vi "Example.vi"() -> ()   [LabVIEW 2020, in "lvpptx.lvlib"]
uses:
  lvpptx.lvlib
  Font.ctl
  Textframe Resize Policy.ctl
  Slide Type.ctl
  Position.ctl
  Size.ctl
panel:
  in  "Text":string
  in  "Text formatting":T1={"Font"="Arial", "Size"=18.0, "Italic"=FALSE, "Bold"=FALSE, "Underline"=FALSE, "Color"=0}
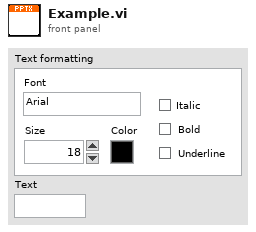
[diagram p1: front panel]
types:
  T1 = typedef "lvpptx.lvlib/Font.ctl" = cluster{"Font":string, "Size":dbl, "Italic":bool, "Bold":bool, "Underline":bool, "Color":u32}
  T2 = typedef "lvpptx.lvlib/Size.ctl" = cluster{"W":dbl, "H":dbl}
  T3 = typedef "lvpptx.lvlib/Position.ctl" = cluster{"X":dbl, "Y":dbl}
  T4 = typedef "lvpptx.lvlib/Slide Type.ctl" = i32
  T5 = typedef "Textframe Resize Policy.ctl" = enum16{"Do not resize", "Expand horizontally", "Expand vertically"}
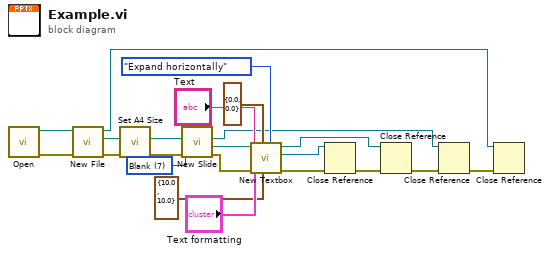
[diagram p0: block diagram]
diagram:
  w11 = T4 7 items=["Title Slide"=1, "Title and Content"=2, "Section Header"=3, "Two Content"=4, "Comparison"=5, "Title Only"=6, "Blank"=7] ("Type")
  n1 = call "Open.vi"() -> ("error out"=w22:errorcluster, "Refnum"=w21:refnum<k7>)  [unwired: 10 in]
  n2 = call "New File.vi"("error in (no error)"=w22, "Refnum"=w21) -> ("error out"=w19:errorcluster, "File refnum"=w20:refnum<k7>, "App refnum out"=w2:refnum<k7>)  [unwired: 7 in]
  n3 = call "Set A4 Size.vi"("error in (no error)"=w19, "File refnum"=w20) -> ("error out"=w17:errorcluster, "File refnum out"=w18:refnum<k7>)  [unwired: 8 in]
  n4 = call "New Slide.vi"("error in (no error)"=w17, "Type"=w11, "File refnum"=w18) -> ("error out"=w15:errorcluster, "Slide refnum out"=w16:refnum<k7>, "File refnum out"=w4:refnum<k7>)  [unwired: 6 in]
  n5 = call "New Textbox.vi"("Resize policy"=Textframe_Resize_Policy."Expand horizontally", "Size"=T2 {"W"=10.0, "H"=10.0}, "Position"=T3 {"X"=0.0, "Y"=0.0}, "error in (no error)"=w15, "Text formatting"="Text formatting", "Text"="Text", "Slide refnum"=w16) -> ("error out"=w9:errorcluster, "Textbox refnum out"=w8:refnum<k7>, "Slide refnum out"=w6:refnum<k7>)  [unwired: 2 in]
  n6 = Close Reference(reference=w8, error in (no error)=w9) -> (error out=w7:errorcluster)
  n7 = Close Reference(reference=w6, error in (no error)=w7) -> (error out=w5:errorcluster)
  n8 = Close Reference(reference=w4, error in (no error)=w5) -> (error out=w3:errorcluster)
  n9 = Close Reference(reference=w2, error in (no error)=w3) -> ()  [unwired: 1 out]
